vi "DPointGrayG3.vi"() -> ()   [LabVIEW 2011]
uses:
  <vilib>/vision/Image Controls.llb/IMAQ Image.ctl
  <vilib>/vision/driver/IMAQdx.llb/IMAQdx Camera Control Mode.ctl
  <vilib>/vision/driver/IMAQdx.llb/IMAQdx Attribute Type.ctl
  <vilib>/vision/driver/IMAQdx.llb/IMAQdx Buffer Number Mode.ctl
  <vilib>/vision/driver/IMAQdx.llb/IMAQdx Acquisition Mode.ctl
  <vilib>/vision/driver/NI_Vision_Acquisition_Software.lvlib
  National Instruments/LabVIEW 2011/resource/objmgr/imaqdx.rc
panel:
  out "String":string="cam0"
  out "binning":i32=1
  out "save all?":bool
  out "image":i32
  out "run":i32
  out "error":errorcluster
  # "Tested with GS3-U3-23S6\nIn M&A-Explorer:\nright click cam, Driver\nselect NI-IMAQdx ..USB3\nand test camera there\nexposure time is not correct\ndid not found the units 1µs?"
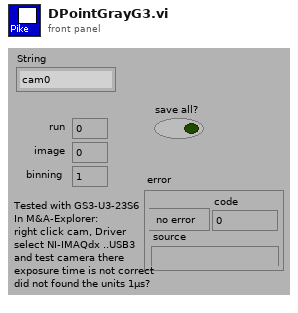
[diagram p1: front panel]
types:
  T1 = typedef "NI_Vision_Acquisition_Software.lvlib/IMAQdx Attribute Type.ctl" = enum32{"U32", "I64", "DBL", "String", "Enum", "Bool", "Command"}
  T2 = cluster{"Attribute Name":string, "Attribute Type":T1, "Value":string}[]
  T3 = cluster{"Attribute Type":T1, "Readable":bool, "Writable":bool, "Attribute Name":string, "Value":string}[]
  T4 = enum16{"None/#Datasets", "Clear", "TagValueOf#", "AddValues", "ReadValue", "ChangeValue", "Get all"}
  T5 = typedef "NI_Vision_Acquisition_Software.lvlib/IMAQdx Camera Control Mode.ctl" = enum32{"Controller", "Listener"}
  T6 = typedef "IMAQ Image.ctl" = refnum<image>
  T7 = cluster{"Type":u32, "Version":u32, "Flags":u32, "SerialNumberHigh":u32, "SerialNumberLow":u32, "BusType":u32, "InterfaceName":string, "VendorName":string, "ModelName":string, "CameraFileName":string, "CameraAttributeURL":string}[]
  T8 = typedef "IMAQdx.ctl" = refnum<k21>
  T9 = cluster{"Center":cluster{dbl, dbl}, "Rotate (rad)":dbl, "MirrorY":bool, "Scale":dbl}
  T10 = enum16{"status", "createIMAQ", "getIMAQ", "getNumber", "deleteIMAQ", "deleteAll", "MemoryUsage", "GetAccess", "DecreaseAccess", "ActualIndex", "ElementToNumber"}
  T11 = enum16{"status", "saveMeta", "getMeta", "deleteMeta", "deleteAll", "MemoryUsage"}
  T12 = typedef "NI_Vision_Acquisition_Software.lvlib/IMAQdx Buffer Number Mode.ctl" = enum32{"Next", "Last", "Buffer Number"}
  T13 = typedef "NI_Vision_Acquisition_Software.lvlib/IMAQdx Acquisition Mode.ctl" = enum32{"One Shot", "Continuous"}
  T14 = enum16{"status", "createIMAQ", "getIMAQ", "getNumber", "deleteIMAQ", "deleteAll", "MemoryUsage", "GetAccess", "DecreaseAccess", "ActualIndex"}
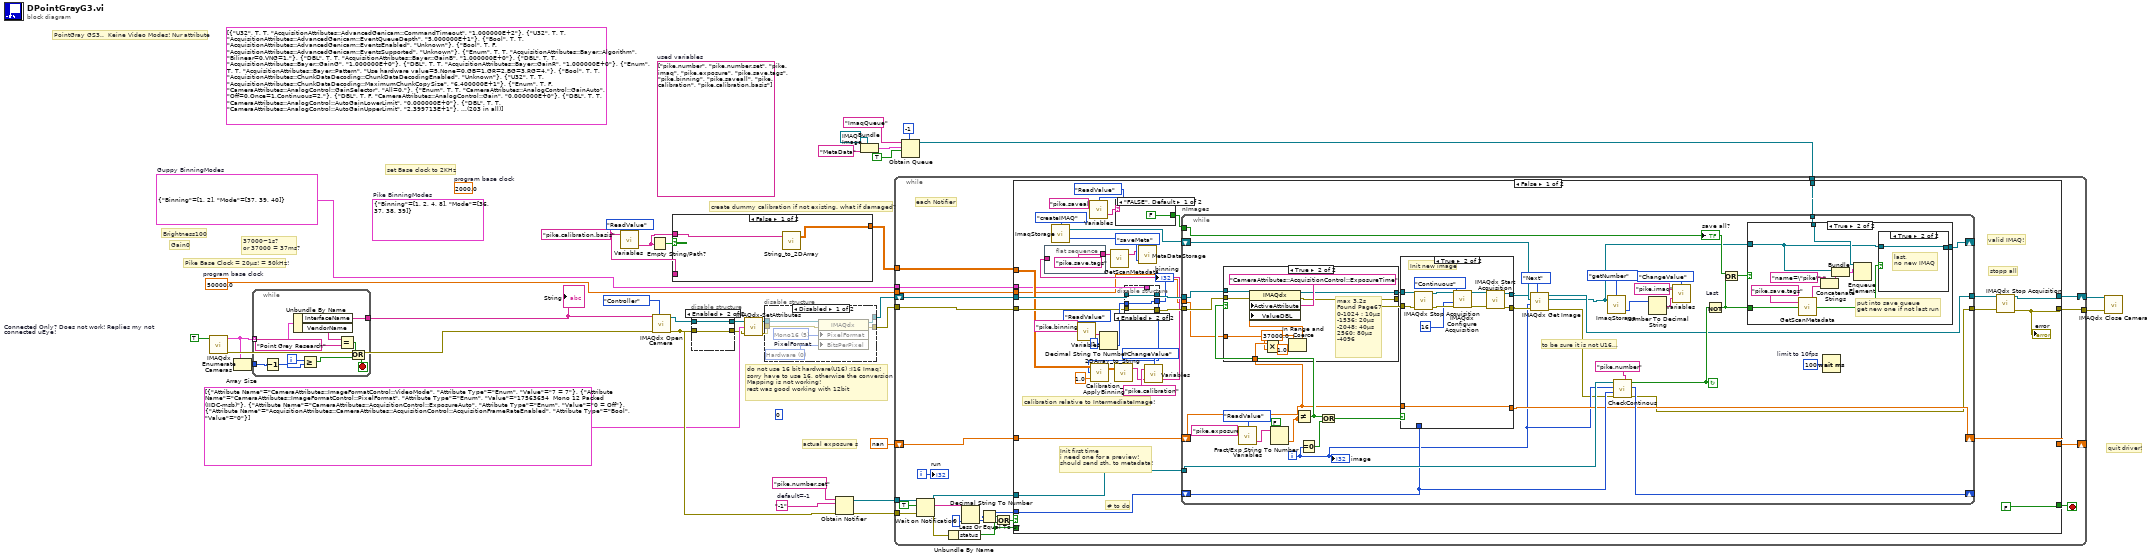
[diagram p0: block diagram]
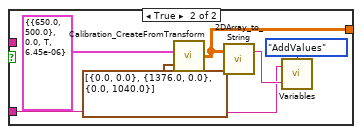
[diagram p3: hidden frame]
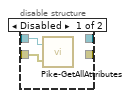
[diagram p4: hidden frame]
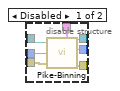
[diagram p5: hidden frame]
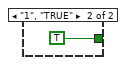
[diagram p6: hidden frame]
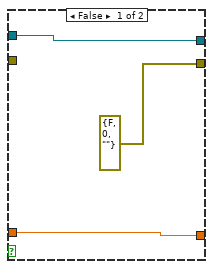
[diagram p8: hidden frame]
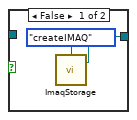
[diagram p10: hidden frame]
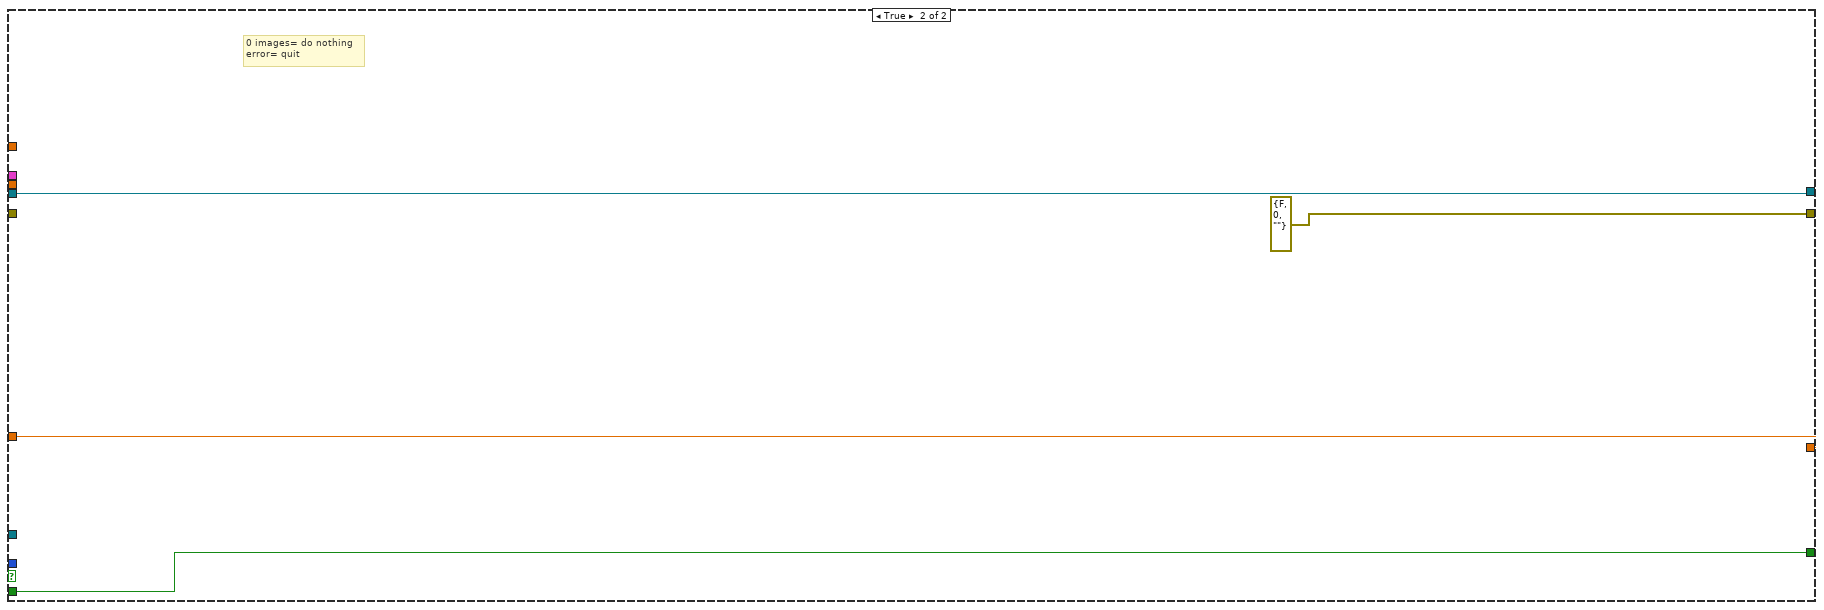
[diagram p11: hidden frame]
diagram:
  (unwired) u32 0 ("PixelFormat")
  (unwired) T3 [{"Attribute Type"=enum."U32", "Readable"=TRUE, "Writable"=TRUE, "Attribute Name"="AcquisitionAttributes::AdvancedGenicam::CommandTimeout", "Value"="1.000000E+2"}, {"Attribute Type"=enum."U32", "Readable"=TRUE, "Writable"=TRUE, "Attribute Name"="AcquisitionAttributes::AdvancedGenicam::EventQueueDepth", "Value"="5.000000E+1"}, {"Attribute Type"=enum."Bool", "Readable"=TRUE, "Writable"=TRUE, "Attribute Name"="AcquisitionAttributes::AdvancedGenicam::EventsEnabled", "Value"="Unknown"}, {"Attribute Type"=enum."Bool", "Readable"=TRUE, "Writable"=FALSE, "Attribute Name"="AcquisitionAttributes::AdvancedGenicam::EventsSupported", "Value"="Unknown"}, {"Attribute Type"=enum."Enum", "Readable"=TRUE, "Writable"=TRUE, "Attribute Name"="AcquisitionAttributes::Bayer::Algorithm", "Value"="Bilinear=0,VNG=1,"}, {"Attribute Type"=enum."DBL", "Readable"=TRUE, "Writable"=TRUE, "Attribute Name"="AcquisitionAttributes::Bayer::GainB", "Value"="1.000000E+0"}, {"Attribute Type"=enum."DBL", "Readable"=TRUE, "Writable"=TRUE, "Attribute Name"="AcquisitionAttributes::Bayer::GainG", "Value"="1.000000E+0"}, {"Attribute Type"=enum."DBL", "Readable"=TRUE, "Writable"=TRUE, "Attribute Name"="AcquisitionAttributes::Bayer::GainR", "Value"="1.000000E+0"}, {"Attribute Type"=enum."Enum", "Readable"=TRUE, "Writable"=TRUE, "Attribute Name"="AcquisitionAttributes::Bayer::Pattern", "Value"="Use hardware value=5,None=0,GB=1,GR=2,BG=3,RG=4,"}, {"Attribute Type"=enum."Bool", "Readable"=TRUE, "Writable"=TRUE, "Attribute Name"="AcquisitionAttributes::ChunkDataDecoding::ChunkDataDecodingEnabled", "Value"="Unknown"}, {"Attribute Type"=enum."U32", "Readable"=TRUE, "Writable"=TRUE, "Attribute Name"="AcquisitionAttributes::ChunkDataDecoding::MaximumChunkCopySize", "Value"="6.400000E+1"}, {"Attribute Type"=enum."Enum", "Readable"=TRUE, "Writable"=FALSE, "Attribute Name"="CameraAttributes::AnalogControl::GainSelector", "Value"="All=0,"}, {"Attribute Type"=enum."Enum", "Readable"=TRUE, "Writable"=TRUE, "Attribute Name"="CameraAttributes::AnalogControl::GainAuto", "Value"="Off=0,Once=1,Continuous=2,"}, {"Attribute Type"=enum."DBL", "Readable"=TRUE, "Writable"=FALSE, "Attribute Name"="CameraAttributes::AnalogControl::Gain", "Value"="0.000000E+0"}, {"Attribute Type"=enum."DBL", "Readable"=TRUE, "Writable"=TRUE, "Attribute Name"="CameraAttributes::AnalogControl::AutoGainLowerLimit", "Value"="0.000000E+0"}, {"Attribute Type"=enum."DBL", "Readable"=TRUE, "Writable"=TRUE, "Attribute Name"="CameraAttributes::AnalogControl::AutoGainUpperLimit", "Value"="2.399713E+1"}, {"Attribute Type"=enum."DBL", "Readable"=TRUE, "Writable"=TRUE, "Attribute Name"="CameraAttributes::AnalogControl::BlackLevel", "Value"="2.709961E+0"}, {"Attribute Type"=enum."Bool", "Readable"=TRUE, "Writable"=TRUE, "Attribute Name"="CameraAttributes::AnalogControl::BlackLevelEnabled", "Value"="Unknown"}, {"Attribute Type"=enum."DBL", "Readable"=TRUE, "Writable"=TRUE, "Attribute Name"="CameraAttributes::AnalogControl::Gamma", "Value"="1.250000E+0"}, {"Attribute Type"=enum."Bool", "Readable"=TRUE, "Writable"=TRUE, "Attribute Name"="CameraAttributes::AnalogControl::GammaEnabled", "Value"="Unknown"}, {"Attribute Type"=enum."I64", "Readable"=TRUE, "Writable"=FALSE, "Attribute Name"="CameraAttributes::AnalogControl::Sharpness", "Value"="1.534000E+3"}, {"Attribute Type"=enum."Bool", "Readable"=TRUE, "Writable"=TRUE, "Attribute Name"="CameraAttributes::AnalogControl::SharpnessEnabled", "Value"="Unknown"}, {"Attribute Type"=enum."Enum", "Readable"=TRUE, "Writable"=TRUE, "Attribute Name"="CameraAttributes::AnalogControl::SharpnessAuto", "Value"="Off=0,Continuous=2,"}, {"Attribute Type"=enum."Bool", "Readable"=FALSE, "Writable"=FALSE, "Attribute Name"="CameraAttributes::AnalogControl::HueEnabled", "Value"="Unknown"}, {"Attribute Type"=enum."Bool", "Readable"=FALSE, "Writable"=FALSE, "Attribute Name"="CameraAttributes::AnalogControl::SaturationEnabled", "Value"="Unknown"}, {"Attribute Type"=enum."String", "Readable"=TRUE, "Writable"=FALSE, "Attribute Name"="CameraAttributes::DeviceControl::DeviceVendorName", "Value"="Point Grey Research"}, {"Attribute Type"=enum."String", "Readable"=TRUE, "Writable"=FALSE, "Attribute Name"="CameraAttributes::DeviceControl::DeviceModelName", "Value"="Grasshopper3 GS3-U3-23S6M"}, {"Attribute Type"=enum."String", "Readable"=TRUE, "Writable"=FALSE, "Attribute Name"="CameraAttributes::DeviceControl::DeviceVersion", "Value"="FW:v2.7.3.00 FPGA:v2.02"}, {"Attribute Type"=enum."String", "Readable"=TRUE, "Writable"=FALSE, "Attribute Name"="CameraAttributes::DeviceControl::DeviceSerialNumber", "Value"="14120127"}, {"Attribute Type"=enum."String", "Readable"=TRUE, "Writable"=TRUE, "Attribute Name"="CameraAttributes::DeviceControl::DeviceUserID", "Value"=""}, {"Attribute Type"=enum."I64", "Readable"=TRUE, "Writable"=FALSE, "Attribute Name"="CameraAttributes::DeviceControl::DeviceGenCpVersionMajor", "Value"="1.000000E+0"}, {"Attribute Type"=enum."I64", "Readable"=TRUE, "Writable"=FALSE, "Attribute Name"="CameraAttributes::DeviceControl::DeviceGenCPVersionMinor", "Value"="0.000000E+0"}, {"Attribute Type"=enum."String", "Readable"=TRUE, "Writable"=FALSE, "Attribute Name"="CameraAttributes::DeviceControl::DeviceFamilyName", "Value"="GEN2-USB"}, {"Attribute Type"=enum."Bool", "Readable"=TRUE, "Writable"=FALSE, "Attribute Name"="CameraAttributes::DeviceControl::U3VDeviceCapability::UserNameAvailable", "Value"="Unknown"}, {"Attribute Type"=enum."Bool", "Readable"=TRUE, "Writable"=FALSE, "Attribute Name"="CameraAttributes::DeviceControl::U3VDeviceCapability::AccessPrivilegeAvailable", "Value"="Unknown"}, {"Attribute Type"=enum."Bool", "Readable"=TRUE, "Writable"=FALSE, "Attribute Name"="CameraAttributes::DeviceControl::U3VDeviceCapability::MessageChannelSupported", "Value"="Unknown"}, {"Attribute Type"=enum."Bool", "Readable"=TRUE, "Writable"=FALSE, "Attribute Name"="CameraAttributes::DeviceControl::U3VDeviceCapability::TimestampSupported", "Value"="Unknown"}, {"Attribute Type"=enum."I64", "Readable"=TRUE, "Writable"=FALSE, "Attribute Name"="CameraAttributes::DeviceControl::U3VDeviceCapability::StringEncoding", "Value"="0.000000E+0"}, {"Attribute Type"=enum."Bool", "Readable"=TRUE, "Writable"=FALSE, "Attribute Name"="CameraAttributes::DeviceControl::U3VDeviceCapability::FamilyRegisterAvailable", "Value"="Unknown"}, {"Attribute Type"=enum."Bool", "Readable"=TRUE, "Writable"=FALSE, "Attribute Name"="CameraAttributes::DeviceControl::U3VDeviceCapability::SBRMSupported", "Value"="Unknown"}, {"Attribute Type"=enum."Bool", "Readable"=TRUE, "Writable"=FALSE, "Attribute Name"="CameraAttributes::DeviceControl::U3VDeviceCapability::EndianessRegistersSupported", "Value"="Unknown"}, {"Attribute Type"=enum."Bool", "Readable"=TRUE, "Writable"=FALSE, "Attribute Name"="CameraAttributes::DeviceControl::U3VDeviceCapability::WrittenLengthFieldSupported", "Value"="Unknown"}, {"Attribute Type"=enum."I64", "Readable"=TRUE, "Writable"=FALSE, "Attribute Name"="CameraAttributes::DeviceControl::Timestamp", "Value"="0.000000E+0"}, {"Attribute Type"=enum."Command", "Readable"=FALSE, "Writable"=TRUE, "Attribute Name"="CameraAttributes::DeviceControl::TimestampLatch", "Value"="Unknown"}, {"Attribute Type"=enum."I64", "Readable"=TRUE, "Writable"=FALSE, "Attribute Name"="CameraAttributes::DeviceControl::TimestampIncrement", "Value"="1.250000E+5"}, {"Attribute Type"=enum."String", "Readable"=TRUE, "Writable"=FALSE, "Attribute Name"="CameraAttributes::DeviceControl::pgrSensorDescription", "Value"="Sony IMX174 (1/1.2\" Mono CMOS)"}, {"Attribute Type"=enum."String", "Readable"=TRUE, "Writable"=FALSE, "Attribute Name"="CameraAttributes::DeviceControl::DeviceSVNVersion", "Value"="FW:0 FPGA:0"}, {"Attribute Type"=enum."String", "Readable"=TRUE, "Writable"=FALSE, "Attribute Name"="CameraAttributes::DeviceControl::DeviceFirmwareVersion", "Value"="2.7.3.00"}, {"Attribute Type"=enum."Enum", "Readable"=TRUE, "Writable"=FALSE, "Attribute Name"="CameraAttributes::DeviceControl::DeviceScanType", "Value"="Areascan=0,"}, {"Attribute Type"=enum."DBL", "Readable"=TRUE, "Writable"=FALSE, "Attribute Name"="CameraAttributes::DeviceControl::DeviceTemperature", "Value"="4.785000E+1"}, {"Attribute Type"=enum."I64", "Readable"=TRUE, "Writable"=FALSE, "Attribute Name"="CameraAttributes::DeviceControl::pgrDeviceUptime", "Value"="9.150000E+2"}, {"Attribute Type"=enum."Enum", "Readable"=TRUE, "Writable"=TRUE, "Attribute Name"="CameraAttributes::DeviceControl::AutoFunctionAOIsControl", "Value"="Off=0,On=1,"}, {"Attribute Type"=enum."I64", "Readable"=FALSE, "Writable"=FALSE, "Attribute Name"="CameraAttributes::DeviceControl::AutoFunctionAOIWidth", "Value"="0.000000E+0"}, {"Attribute Type"=enum."I64", "Readable"=FALSE, "Writable"=FALSE, "Attribute Name"="CameraAttributes::DeviceControl::AutoFunctionAOIHeight", "Value"="0.000000E+0"}, {"Attribute Type"=enum."I64", "Readable"=FALSE, "Writable"=FALSE, "Attribute Name"="CameraAttributes::DeviceControl::AutoFunctionAOIOffsetX", "Value"="0.000000E+0"}, {"Attribute Type"=enum."I64", "Readable"=FALSE, "Writable"=FALSE, "Attribute Name"="CameraAttributes::DeviceControl::AutoFunctionAOIOffsetY", "Value"="0.000000E+0"}, {"Attribute Type"=enum."Enum", "Readable"=TRUE, "Writable"=TRUE, "Attribute Name"="CameraAttributes::DeviceControl::pgrDevicePowerSupplySelector", "Value"="External=0,LinkPower=1,5.0 Volts=2,Sensor Power=6,"}, {"Attribute Type"=enum."Enum", "Readable"=TRUE, "Writable"=FALSE, "Attribute Name"="CameraAttributes::DeviceControl::pgrPowerSourcePresent", "Value"="False=0,True=1,"}, {"Attribute Type"=enum."Enum", "Readable"=FALSE, "Writable"=FALSE, "Attribute Name"="CameraAttributes::DeviceControl::pgrPowerSupplyEnable", "Value"="False=0,True=1,"}, {"Attribute Type"=enum."DBL", "Readable"=TRUE, "Writable"=FALSE, "Attribute Name"="CameraAttributes::DeviceControl::pgrPowerSupplyVoltage", "Value"="0.000000E+0"}, {"Attribute Type"=enum."DBL", "Readable"=TRUE, "Writable"=FALSE, "Attribute Name"="CameraAttributes::DeviceControl::pgrPowerSupplyCurrent", "Value"="6.889992E-1"}, {"Attribute Type"=enum."I64", "Readable"=TRUE, "Writable"=FALSE, "Attribute Name"="CameraAttributes::DeviceControl::DeviceMaxThroughput", "Value"="3.041280E+8"}, {"Attribute Type"=enum."I64", "Readable"=TRUE, "Writable"=TRUE, "Attribute Name"="CameraAttributes::DeviceControl::DeviceLinkThroughputLimit", "Value"="3.041280E+8"}, {"Attribute Type"=enum."Enum", "Readable"=TRUE, "Writable"=TRUE, "Attribute Name"="CameraAttributes::AcquisitionControl::TriggerSelector", "Value"="Frame Start=0,Exposure Active=1,"}, {"Attribute Type"=enum."Enum", "Readable"=TRUE, "Writable"=TRUE, "Attribute Name"="CameraAttributes::AcquisitionControl::TriggerMode", "Value"="Off=0,On=1,"}, {"Attribute Type"=enum."Command", "Readable"=FALSE, "Writable"=FALSE, "Attribute Name"="CameraAttributes::AcquisitionControl::TriggerSoftware", "Value"="Unknown"}, {"Attribute Type"=enum."Enum", "Readable"=TRUE, "Writable"=TRUE, "Attribute Name"="CameraAttributes::AcquisitionControl::TriggerSource", "Value"="Software=7,Line 0=0,Line 2=2,Line 3=3,"}, {"Attribute Type"=enum."Enum", "Readable"=TRUE, "Writable"=TRUE, "Attribute Name"="CameraAttributes::AcquisitionControl::TriggerActivation", "Value"="Rising Edge=1,Falling Edge=0,"}, {"Attribute Type"=enum."DBL", "Readable"=TRUE, "Writable"=TRUE, "Attribute Name"="CameraAttributes::AcquisitionControl::TriggerDelay", "Value"="0.000000E+0"}, {"Attribute Type"=enum."Bool", "Readable"=TRUE, "Writable"=TRUE, "Attribute Name"="CameraAttributes::AcquisitionControl::TriggerDelayEnabled", "Value"="Unknown"}, {"Attribute Type"=enum."Enum", "Readable"=TRUE, "Writable"=TRUE, "Attribute Name"="CameraAttributes::AcquisitionControl::ExposureMode", "Value"="Timed=0,Trigger Width=1,"}, {"Attribute Type"=enum."Enum", "Readable"=TRUE, "Writable"=TRUE, "Attribute Name"="CameraAttributes::AcquisitionControl::ExposureAuto", "Value"="Off=0,Once=1,Continuous=2,"}, {"Attribute Type"=enum."DBL", "Readable"=TRUE, "Writable"=FALSE, "Attribute Name"="CameraAttributes::AcquisitionControl::ExposureTime", "Value"="2.435267E+3"}, {"Attribute Type"=enum."DBL", "Readable"=TRUE, "Writable"=TRUE, "Attribute Name"="CameraAttributes::AcquisitionControl::AutoExposureTimeLowerLimit", "Value"="9.119511E+0"}, {"Attribute Type"=enum."DBL", "Readable"=TRUE, "Writable"=TRUE, "Attribute Name"="CameraAttributes::AcquisitionControl::AutoExposureTimeUpperLimit", "Value"="1.152647E+4"}, {"Attribute Type"=enum."Enum", "Readable"=TRUE, "Writable"=TRUE, "Attribute Name"="CameraAttributes::AcquisitionControl::pgrExposureCompensationAuto", "Value"="Off=0,Once=1,Continuous=2,"}, {"Attribute Type"=enum."DBL", "Readable"=TRUE, "Writable"=FALSE, "Attribute Name"="CameraAttributes::AcquisitionControl::pgrExposureCompensation", "Value"="6.629639E-1"}, {"Attribute Type"=enum."DBL", "Readable"=TRUE, "Writable"=TRUE, "Attribute Name"="CameraAttributes::AcquisitionControl::pgrAutoExposureCompensationLowerLimit", "Value"="4.150391E-1"}, {"Attribute Type"=enum."DBL", "Readable"=TRUE, "Writable"=TRUE, "Attribute Name"="CameraAttributes::AcquisitionControl::pgrAutoExposureCompensationUpperLimit", "Value"="2.000000E+0"}, {"Attribute Type"=enum."Enum", "Readable"=TRUE, "Writable"=TRUE, "Attribute Name"="CameraAttributes::AcquisitionControl::AcquisitionMode", "Value"="Continuous=0,SingleFrame=1,MultiFrame=2,"}, {"Attribute Type"=enum."Enum", "Readable"=TRUE, "Writable"=TRUE, "Attribute Name"="CameraAttributes::AcquisitionControl::AcquisitionFrameRateAuto", "Value"="Off=0,Continuous=2,"}, {"Attribute Type"=enum."Bool", "Readable"=TRUE, "Writable"=TRUE, "Attribute Name"="CameraAttributes::AcquisitionControl::AcquisitionFrameRateEnabled", "Value"="Unknown"}, {"Attribute Type"=enum."DBL", "Readable"=TRUE, "Writable"=FALSE, "Attribute Name"="CameraAttributes::AcquisitionControl::AcquisitionFrameRate", "Value"="8.600000E+1"}, {"Attribute Type"=enum."I64", "Readable"=FALSE, "Writable"=FALSE, "Attribute Name"="CameraAttributes::AcquisitionControl::AcquisitionFrameCount", "Value"="0.000000E+0"}, {"Attribute Type"=enum."Enum", "Readable"=TRUE, "Writable"=TRUE, "Attribute Name"="CameraAttributes::ImageFormatControl::PixelFormat", "Value"="Mono 8=17301505,Mono 12 Packed (IIDC-msb)=17563654,Mono 12 Packed=17563719,Mono 16=17825799,"}, {"Attribute Type"=enum."Bool", "Readable"=TRUE, "Writable"=TRUE, "Attribute Name"="CameraAttributes::ImageFormatControl::OnBoardColorProcessEnabled", "Value"="Unknown"}, {"Attribute Type"=enum."I64", "Readable"=TRUE, "Writable"=TRUE, "Attribute Name"="CameraAttributes::ImageFormatControl::Width", "Value"="1.920000E+3"}, {"Attribute Type"=enum."I64", "Readable"=TRUE, "Writable"=TRUE, "Attribute Name"="CameraAttributes::ImageFormatControl::Height", "Value"="1.200000E+3"}, {"Attribute Type"=enum."I64", "Readable"=TRUE, "Writable"=TRUE, "Attribute Name"="CameraAttributes::ImageFormatControl::OffsetX", "Value"="0.000000E+0"}, {"Attribute Type"=enum."I64", "Readable"=TRUE, "Writable"=TRUE, "Attribute Name"="CameraAttributes::ImageFormatControl::OffsetY", "Value"="0.000000E+0"}, {"Attribute Type"=enum."I64", "Readable"=TRUE, "Writable"=FALSE, "Attribute Name"="CameraAttributes::ImageFormatControl::SensorWidth", "Value"="1.920000E+3"}, {"Attribute Type"=enum."I64", "Readable"=TRUE, "Writable"=FALSE, "Attribute Name"="CameraAttributes::ImageFormatControl::SensorHeight", "Value"="1.200000E+3"}, {"Attribute Type"=enum."I64", "Readable"=TRUE, "Writable"=FALSE, "Attribute Name"="CameraAttributes::ImageFormatControl::WidthMax", "Value"="1.920000E+3"}, {"Attribute Type"=enum."I64", "Readable"=TRUE, "Writable"=FALSE, "Attribute Name"="CameraAttributes::ImageFormatControl::HeightMax", "Value"="1.200000E+3"}, {"Attribute Type"=enum."Enum", "Readable"=TRUE, "Writable"=TRUE, "Attribute Name"="CameraAttributes::ImageFormatControl::VideoMode", "Value"="0=0,1=1,7=7,"}, {"Attribute Type"=enum."I64", "Readable"=TRUE, "Writable"=FALSE, "Attribute Name"="CameraAttributes::ImageFormatControl::BinningHorizontal", "Value"="1.000000E+0"}, {"Attribute Type"=enum."I64", "Readable"=TRUE, "Writable"=TRUE, "Attribute Name"="CameraAttributes::ImageFormatControl::BinningVertical", "Value"="1.000000E+0"}, {"Attribute Type"=enum."Bool", "Readable"=TRUE, "Writable"=TRUE, "Attribute Name"="CameraAttributes::ImageFormatControl::ReverseX", "Value"="Unknown"}, {"Attribute Type"=enum."Enum", "Readable"=TRUE, "Writable"=FALSE, "Attribute Name"="CameraAttributes::ImageFormatControl::PixelSize", "Value"="8 Bits/Pixel=8,10 Bits/Pixel=10,12 Bits/Pixel=12,16 Bits/Pixel=16,24 Bits/Pixel=24,32 Bits/Pixel=32,"}, {"Attribute Type"=enum."Enum", "Readable"=TRUE, "Writable"=FALSE, "Attribute Name"="CameraAttributes::ImageFormatControl::PixelColorFilter", "Value"="BayerRG=0,BayerGB=1,BayerGR=2,BayerBG=3,None=255,"}, {"Attribute Type"=enum."I64", "Readable"=TRUE, "Writable"=FALSE, "Attribute Name"="CameraAttributes::ImageFormatControl::PixelDynamicRangeMin", "Value"="0.000000E+0"}, {"Attribute Type"=enum."I64", "Readable"=TRUE, "Writable"=FALSE, "Attribute Name"="CameraAttributes::ImageFormatControl::PixelDynamicRangeMax", "Value"="0.000000E+0"}, {"Attribute Type"=enum."Enum", "Readable"=TRUE, "Writable"=TRUE, "Attribute Name"="CameraAttributes::ImageFormatControl::TestPattern", "Value"="Off=0,Test Image 1=1,Test Image 2=2,"}, {"Attribute Type"=enum."Enum", "Readable"=TRUE, "Writable"=FALSE, "Attribute Name"="CameraAttributes::ImageFormatControl::PixelDefectControl::pgrDefectPixelCorrectionType", "Value"="FPGA Correction=0,Sensor Correction=1,"}, {"Attribute Type"=enum."Bool", "Readable"=TRUE, "Writable"=TRUE, "Attribute Name"="CameraAttributes::ImageFormatControl::PixelDefectControl::pgrDefectPixelCorrectionEnable", "Value"="Unknown"}, {"Attribute Type"=enum."Enum", "Readable"=TRUE, "Writable"=TRUE, "Attribute Name"="CameraAttributes::ImageFormatControl::PixelDefectControl::pgrDefectPixelCorrectionTestMode", "Value"="Off=0,On=1,"}, {"Attribute Type"=enum."I64", "Readable"=TRUE, "Writable"=TRUE, "Attribute Name"="CameraAttributes::ImageFormatControl::PixelDefectControl::pgrCurrentCorrectedPixelCount", "Value"="6.000000E+0"}, {"Attribute Type"=enum."I64", "Readable"=TRUE, "Writable"=TRUE, "Attribute Name"="CameraAttributes::ImageFormatControl::PixelDefectControl::pgrCurrentCorrectedPixelIndex", "Value"="0.000000E+0"}, {"Attribute Type"=enum."I64", "Readable"=TRUE, "Writable"=TRUE, "Attribute Name"="CameraAttributes::ImageFormatControl::PixelDefectControl::pgrCurrentCorrectedPixelOffsetX", "Value"="1.151000E+3"}, {"Attribute Type"=enum."I64", "Readable"=TRUE, "Writable"=TRUE, "Attribute Name"="CameraAttributes::ImageFormatControl::PixelDefectControl::pgrCurrentCorrectedPixelOffsetY", "Value"="5.900000E+1"}, {"Attribute Type"=enum."Command", "Readable"=FALSE, "Writable"=TRUE, "Attribute Name"="CameraAttributes::ImageFormatControl::PixelDefectControl::pgrCurrentCorrectedPixelSave", "Value"="Unknown"}, {"Attribute Type"=enum."I64", "Readable"=TRUE, "Writable"=FALSE, "Attribute Name"="CameraAttributes::UserSetControl::UserSetCurrent", "Value"="0.000000E+0"}, {"Attribute Type"=enum."Enum", "Readable"=TRUE, "Writable"=TRUE, "Attribute Name"="CameraAttributes::UserSetControl::UserSetSelector", "Value"="Default=0,User Set 1=1,User Set 2=2,"}, {"Attribute Type"=enum."Command", "Readable"=FALSE, "Writable"=TRUE, "Attribute Name"="CameraAttributes::UserSetControl::UserSetLoad", "Value"="Unknown"}, {"Attribute Type"=enum."Command", "Readable"=FALSE, "Writable"=TRUE, "Attribute Name"="CameraAttributes::UserSetControl::UserSetSave", "Value"="Unknown"}, {"Attribute Type"=enum."Enum", "Readable"=TRUE, "Writable"=TRUE, "Attribute Name"="CameraAttributes::UserSetControl::UserSetDefault", "Value"="Default=0,User Set 1=1,User Set 2=2,"}, {"Attribute Type"=enum."I64", "Readable"=TRUE, "Writable"=FALSE, "Attribute Name"="CameraAttributes::DataFlashControl::DataFlashPageSize", "Value"="2.560000E+2"}, {"Attribute Type"=enum."I64", "Readable"=TRUE, "Writable"=FALSE, "Attribute Name"="CameraAttributes::DataFlashControl::DataFlashPageCount", "Value"="8.192000E+3"}, {"Attribute Type"=enum."I64", "Readable"=TRUE, "Writable"=TRUE, "Attribute Name"="CameraAttributes::DataFlashControl::ActivePageNumber", "Value"="0.000000E+0"}, {"Attribute Type"=enum."I64", "Readable"=TRUE, "Writable"=TRUE, "Attribute Name"="CameraAttributes::DataFlashControl::ActivePageOffset", "Value"="0.000000E+0"}, {"Attribute Type"=enum."I64", "Readable"=TRUE, "Writable"=TRUE, "Attribute Name"="CameraAttributes::DataFlashControl::ActivePageValue", "Value"="1.129859E+9"}, {"Attribute Type"=enum."Command", "Readable"=FALSE, "Writable"=TRUE, "Attribute Name"="CameraAttributes::DataFlashControl::ActivePageSave", "Value"="Unknown"}, {"Attribute Type"=enum."Enum", "Readable"=TRUE, "Writable"=TRUE, "Attribute Name"="CameraAttributes::DigitalIOControl::LineSelector", "Value"="Line 0=0,Line 1=1,Line 2=2,Line 3=3,"}, {"Attribute Type"=enum."Enum", "Readable"=TRUE, "Writable"=TRUE, "Attribute Name"="CameraAttributes::DigitalIOControl::LineMode", "Value"="Input=0,Trigger=2,"}, {"Attribute Type"=enum."Enum", "Readable"=FALSE, "Writable"=FALSE, "Attribute Name"="CameraAttributes::DigitalIOControl::LineSource", "Value"="ExposureActive=0,ExternalTriggerActive=1,"}, {"Attribute Type"=enum."Bool", "Readable"=FALSE, "Writable"=FALSE, "Attribute Name"="CameraAttributes::DigitalIOControl::LineInverter", "Value"="Unknown"}, {"Attribute Type"=enum."Bool", "Readable"=FALSE, "Writable"=FALSE, "Attribute Name"="CameraAttributes::DigitalIOControl::StrobeEnabled", "Value"="Unknown"}, {"Attribute Type"=enum."DBL", "Readable"=FALSE, "Writable"=FALSE, "Attribute Name"="CameraAttributes::DigitalIOControl::StrobeDelay", "Value"="0.000000E+0"}, {"Attribute Type"=enum."DBL", "Readable"=FALSE, "Writable"=FALSE, "Attribute Name"="CameraAttributes::DigitalIOControl::StrobeDuration", "Value"="0.000000E+0"}, {"Attribute Type"=enum."Bool", "Readable"=FALSE, "Writable"=FALSE, "Attribute Name"="CameraAttributes::DigitalIOControl::UserOutputValue", "Value"="Unknown"}, {"Attribute Type"=enum."I64", "Readable"=TRUE, "Writable"=TRUE, "Attribute Name"="CameraAttributes::DigitalIOControl::LineDebouncerTimeRaw", "Value"="0.000000E+0"}, {"Attribute Type"=enum."Bool", "Readable"=TRUE, "Writable"=FALSE, "Attribute Name"="CameraAttributes::DigitalIOControl::LineStatus", "Value"="Unknown"}, {"Attribute Type"=enum."I64", "Readable"=TRUE, "Writable"=FALSE, "Attribute Name"="CameraAttributes::DigitalIOControl::LineStatusAll", "Value"="1.400000E+1"}, {"Attribute Type"=enum."I64", "Readable"=TRUE, "Writable"=TRUE, "Attribute Name"="CameraAttributes::TransportLayerControl::U3VMessageChannelID", "Value"="0.000000E+0"}, {"Attribute Type"=enum."I64", "Readable"=TRUE, "Writable"=FALSE, "Attribute Name"="CameraAttributes::TransportLayerControl::U3VVersionMajor", "Value"="1.000000E+0"}, {"Attribute Type"=enum."I64", "Readable"=TRUE, "Writable"=FALSE, "Attribute Name"="CameraAttributes::TransportLayerControl::U3VVersionMinor", "Value"="0.000000E+0"}, {"Attribute Type"=enum."I64", "Readable"=TRUE, "Writable"=FALSE, "Attribute Name"="CameraAttributes::TransportLayerControl::U3VCPCapability", "Value"="0.000000E+0"}, {"Attribute Type"=enum."Bool", "Readable"=TRUE, "Writable"=FALSE, "Attribute Name"="CameraAttributes::TransportLayerControl::U3VCPSIRMAvailable", "Value"="Unknown"}, {"Attribute Type"=enum."Bool", "Readable"=TRUE, "Writable"=FALSE, "Attribute Name"="CameraAttributes::TransportLayerControl::U3VCPEIRMAvailable", "Value"="Unknown"}, {"Attribute Type"=enum."Bool", "Readable"=TRUE, "Writable"=FALSE, "Attribute Name"="CameraAttributes::TransportLayerControl::U3VCPIIDC2Available", "Value"="Unknown"}, {"Attribute Type"=enum."I64", "Readable"=TRUE, "Writable"=FALSE, "Attribute Name"="CameraAttributes::TransportLayerControl::U3VMaxCommandTransferLength", "Value"="1.024000E+3"}, {"Attribute Type"=enum."I64", "Readable"=TRUE, "Writable"=FALSE, "Attribute Name"="CameraAttributes::TransportLayerControl::U3VMaxAcknowledgeTransferLength", "Value"="1.024000E+3"}, {"Attribute Type"=enum."I64", "Readable"=TRUE, "Writable"=FALSE, "Attribute Name"="CameraAttributes::TransportLayerControl::U3VNumberOfStreamChannels", "Value"="1.000000E+0"}, {"Attribute Type"=enum."Enum", "Readable"=TRUE, "Writable"=FALSE, "Attribute Name"="CameraAttributes::TransportLayerControl::U3VCurrentSpeed", "Value"="Low Speed=0,Full Speed=1,High Speed=2,Super Speed=3,"}, {"Attribute Type"=enum."I64", "Readable"=TRUE, "Writable"=FALSE, "Attribute Name"="CameraAttributes::TransportLayerControl::PayloadSize", "Value"="3.456000E+6"}, {"Attribute Type"=enum."I64", "Readable"=TRUE, "Writable"=FALSE, "Attribute Name"="CameraAttributes::TransportLayerControl::TransmitFailureCount", "Value"="0.000000E+0"}, {"Attribute Type"=enum."Command", "Readable"=FALSE, "Writable"=TRUE, "Attribute Name"="CameraAttributes::TransportLayerControl::TransmitFailureCountReset", "Value"="Unknown"}, {"Attribute Type"=enum."I64", "Readable"=TRUE, "Writable"=FALSE, "Attribute Name"="CameraAttributes::TransportLayerControl::USB3LinkRecoveryCount", "Value"="0.000000E+0"}, {"Attribute Type"=enum."Bool", "Readable"=TRUE, "Writable"=TRUE, "Attribute Name"="CameraAttributes::ChunkDataControl::ChunkModeActive", "Value"="Unknown"}, {"Attribute Type"=enum."Enum", "Readable"=TRUE, "Writable"=TRUE, "Attribute Name"="CameraAttributes::ChunkDataControl::ChunkSelector", "Value"="Image CRC=1,Frame Counter=2,Offset X=3,Offset Y=4,Width=5,Height=6,Exposure Time=7,Gain=8,Black Level=9,"}, {"Attribute Type"=enum."Bool", "Readable"=TRUE, "Writable"=TRUE, "Attribute Name"="CameraAttributes::ChunkDataControl::ChunkEnable", "Value"="Unknown"}, {"Attribute Type"=enum."I64", "Readable"=FALSE, "Writable"=FALSE, "Attribute Name"="CameraAttributes::ChunkData::ChunkCRC", "Value"="0.000000E+0"}, {"Attribute Type"=enum."I64", "Readable"=FALSE, "Writable"=FALSE, "Attribute Name"="CameraAttributes::ChunkData::ChunkFrameCounter", "Value"="0.000000E+0"}, {"Attribute Type"=enum."I64", "Readable"=FALSE, "Writable"=FALSE, "Attribute Name"="CameraAttributes::ChunkData::ChunkOffsetX", "Value"="0.000000E+0"}, {"Attribute Type"=enum."I64", "Readable"=FALSE, "Writable"=FALSE, "Attribute Name"="CameraAttributes::ChunkData::ChunkOffsetY", "Value"="0.000000E+0"}, {"Attribute Type"=enum."I64", "Readable"=FALSE, "Writable"=FALSE, "Attribute Name"="CameraAttributes::ChunkData::ChunkWidth", "Value"="0.000000E+0"}, {"Attribute Type"=enum."I64", "Readable"=FALSE, "Writable"=FALSE, "Attribute Name"="CameraAttributes::ChunkData::ChunkHeight", "Value"="0.000000E+0"}, {"Attribute Type"=enum."DBL", "Readable"=FALSE, "Writable"=FALSE, "Attribute Name"="CameraAttributes::ChunkData::ChunkExposureTime", "Value"="0.000000E+0"}, {"Attribute Type"=enum."DBL", "Readable"=FALSE, "Writable"=FALSE, "Attribute Name"="CameraAttributes::ChunkData::ChunkGain", "Value"="0.000000E+0"}, {"Attribute Type"=enum."DBL", "Readable"=FALSE, "Writable"=FALSE, "Attribute Name"="CameraAttributes::ChunkData::ChunkBlackLevel", "Value"="0.000000E+0"}, {"Attribute Type"=enum."Enum", "Readable"=TRUE, "Writable"=TRUE, "Attribute Name"="CameraAttributes::EventControl::EventSelector", "Value"="Acquisition Start=40000,Acquisition End=40001,Exposure Start=40002,Exposure End=40003,"}, {"Attribute Type"=enum."Enum", "Readable"=TRUE, "Writable"=TRUE, "Attribute Name"="CameraAttributes::EventControl::EventNotification", "Value"="On=1,Off=0,"}, {"Attribute Type"=enum."I64", "Readable"=FALSE, "Writable"=FALSE, "Attribute Name"="CameraAttributes::EventControl::EventAcquisitionStartData::EventAcquisitionStart", "Value"="0.000000E+0"}, {"Attribute Type"=enum."I64", "Readable"=FALSE, "Writable"=FALSE, "Attribute Name"="CameraAttributes::EventControl::EventAcquisitionStartData::EventAcquisitionStartTimestamp", "Value"="0.000000E+0"}, {"Attribute Type"=enum."I64", "Readable"=FALSE, "Writable"=FALSE, "Attribute Name"="CameraAttributes::EventControl::EventAcquisitionStartData::EventAcquisitionStartFrameID", "Value"="0.000000E+0"}, {"Attribute Type"=enum."I64", "Readable"=FALSE, "Writable"=FALSE, "Attribute Name"="CameraAttributes::EventControl::EventAcquisitionEndData::EventAcquisitionEnd", "Value"="0.000000E+0"}, {"Attribute Type"=enum."I64", "Readable"=FALSE, "Writable"=FALSE, "Attribute Name"="CameraAttributes::EventControl::EventAcquisitionEndData::EventAcquisitionEndTimestamp", "Value"="0.000000E+0"}, {"Attribute Type"=enum."I64", "Readable"=FALSE, "Writable"=FALSE, "Attribute Name"="CameraAttributes::EventControl::EventAcquisitionEndData::EventAcquisitionEndFrameID", "Value"="0.000000E+0"}, {"Attribute Type"=enum."I64", "Readable"=FALSE, "Writable"=FALSE, "Attribute Name"="CameraAttributes::EventControl::EventExposureStartData::EventExposureStart", "Value"="0.000000E+0"}, {"Attribute Type"=enum."I64", "Readable"=FALSE, "Writable"=FALSE, "Attribute Name"="CameraAttributes::EventControl::EventExposureStartData::EventExposureStartTimestamp", "Value"="0.000000E+0"}, {"Attribute Type"=enum."I64", "Readable"=FALSE, "Writable"=FALSE, "Attribute Name"="CameraAttributes::EventControl::EventExposureStartData::EventExposureStartFrameID", "Value"="0.000000E+0"}, {"Attribute Type"=enum."I64", "Readable"=FALSE, "Writable"=FALSE, "Attribute Name"="CameraAttributes::EventControl::EventExposureEndData::EventExposureEnd", "Value"="0.000000E+0"}, {"Attribute Type"=enum."I64", "Readable"=FALSE, "Writable"=FALSE, "Attribute Name"="CameraAttributes::EventControl::EventExposureEndData::EventExposureEndTimestamp", "Value"="0.000000E+0"}, {"Attribute Type"=enum."I64", "Readable"=FALSE, "Writable"=FALSE, "Attribute Name"="CameraAttributes::EventControl::EventExposureEndData::EventExposureEndFrameID", "Value"="0.000000E+0"}, {"Attribute Type"=enum."Command", "Readable"=FALSE, "Writable"=TRUE, "Attribute Name"="CameraAttributes::EventControl::TriggerEventTest", "Value"="Unknown"}, {"Attribute Type"=enum."I64", "Readable"=FALSE, "Writable"=FALSE, "Attribute Name"="CameraAttributes::EventControl::EventTestData::EventTest", "Value"="0.000000E+0"}, {"Attribute Type"=enum."I64", "Readable"=FALSE, "Writable"=FALSE, "Attribute Name"="CameraAttributes::EventControl::EventTestData::EventTestTimestamp", "Value"="0.000000E+0"}, {"Attribute Type"=enum."I64", "Readable"=FALSE, "Writable"=FALSE, "Attribute Name"="CameraAttributes::EventControl::EventTestData::EventTestFrameID", "Value"="0.000000E+0"}, {"Attribute Type"=enum."Enum", "Readable"=TRUE, "Writable"=TRUE, "Attribute Name"="AcquisitionAttributes::BitsPerPixel", "Value"="Use hardware value=0,10-bit=10,12-bit=12,14-bit=14,16-bit=16,"}, {"Attribute Type"=enum."Enum", "Readable"=TRUE, "Writable"=TRUE, "Attribute Name"="AcquisitionAttributes::ImageDecoderCopyMode", "Value"="Auto=0,Always=1,Never=2,"}, {"Attribute Type"=enum."Enum", "Readable"=TRUE, "Writable"=TRUE, "Attribute Name"="AcquisitionAttributes::IncompleteBufferMode", "Value"="Ignore=0,Fail=1,"}, {"Attribute Type"=enum."Enum", "Readable"=TRUE, "Writable"=TRUE, "Attribute Name"="AcquisitionAttributes::OutputImageType", "Value"="Auto=2147483647,Grayscale (U8)=0,Grayscale (I16)=1,Grayscale (U16)=7,RGB (U32)=4,RGB (U64)=6,"}, {"Attribute Type"=enum."Enum", "Readable"=TRUE, "Writable"=TRUE, "Attribute Name"="AcquisitionAttributes::OverwriteMode", "Value"="Get Oldest=0,Fail=2,Get Newest=3,"}, {"Attribute Type"=enum."Enum", "Readable"=TRUE, "Writable"=TRUE, "Attribute Name"="AcquisitionAttributes::ReceiveTimestampMode", "Value"="None=0,Tick Count=1,System Time=2,"}, {"Attribute Type"=enum."Bool", "Readable"=TRUE, "Writable"=TRUE, "Attribute Name"="AcquisitionAttributes::ShiftPixelBits", "Value"="Unknown"}, {"Attribute Type"=enum."Bool", "Readable"=TRUE, "Writable"=TRUE, "Attribute Name"="AcquisitionAttributes::SwapPixelBytes", "Value"="Unknown"}, {"Attribute Type"=enum."U32", "Readable"=TRUE, "Writable"=TRUE, "Attribute Name"="AcquisitionAttributes::Timeout", "Value"="5.000000E+3"}, {"Attribute Type"=enum."U32", "Readable"=TRUE, "Writable"=FALSE, "Attribute Name"="CameraInformation::BaseAddress", "Value"="0.000000E+0"}, {"Attribute Type"=enum."Enum", "Readable"=TRUE, "Writable"=FALSE, "Attribute Name"="CameraInformation::BusType", "Value"="FireWire=825440564,Ethernet=1768977972,Simulator=544434541,DirectShow=1685284983,IP=1230005101,SmartCamera2=1396924722,USB3 Vision=1431519795,UVC=1431716640,"}, {"Attribute Type"=enum."String", "Readable"=TRUE, "Writable"=FALSE, "Attribute Name"="CameraInformation::ModelName", "Value"="Grasshopper3 GS3-U3-23S6M"}, {"Attribute Type"=enum."String", "Readable"=TRUE, "Writable"=FALSE, "Attribute Name"="CameraInformation::PrimaryURLString", "Value"="Local:Point Grey Research_GEN2-USB_Grasshopper3 GS3-U3-23S6M_FW_v2.7.3.00 FPGA_v2.02_95785afa5ee09562316bc701b412815e5437e6de.zip;00000000fffd0040;0000000000006d52"}, {"Attribute Type"=enum."String", "Readable"=TRUE, "Writable"=FALSE, "Attribute Name"="CameraInformation::SecondaryURLString", "Value"=""}, {"Attribute Type"=enum."U32", "Readable"=TRUE, "Writable"=FALSE, "Attribute Name"="CameraInformation::SerialNumberHigh", "Value"="7.696000E+3"}, {"Attribute Type"=enum."U32", "Readable"=TRUE, "Writable"=FALSE, "Attribute Name"="CameraInformation::SerialNumberLow", "Value"="1.412013E+7"}, {"Attribute Type"=enum."Enum", "Readable"=TRUE, "Writable"=FALSE, "Attribute Name"="CameraInformation::USBConnectionSpeed", "Value"="Low-Speed (USB 2.0)=1,Full-Speed (USB 2.0)=2,Hi-Speed (USB 2.0)=4,SuperSpeed (USB 3.0)=8,"}, {"Attribute Type"=enum."String", "Readable"=TRUE, "Writable"=FALSE, "Attribute Name"="CameraInformation::VendorName", "Value"="Point Grey Research"}, {"Attribute Type"=enum."Bool", "Readable"=TRUE, "Writable"=FALSE, "Attribute Name"="StatusInformation::AcqInProgress", "Value"="Unknown"}, {"Attribute Type"=enum."I64", "Readable"=TRUE, "Writable"=FALSE, "Attribute Name"="StatusInformation::HandledEventCount", "Value"="0.000000E+0"}, {"Attribute Type"=enum."I64", "Readable"=TRUE, "Writable"=FALSE, "Attribute Name"="StatusInformation::IncompleteBufferCount", "Value"="0.000000E+0"}, {"Attribute Type"=enum."I64", "Readable"=TRUE, "Writable"=FALSE, "Attribute Name"="StatusInformation::LastBufferCount", "Value"="0.000000E+0"}, {"Attribute Type"=enum."U32", "Readable"=TRUE, "Writable"=FALSE, "Attribute Name"="StatusInformation::LastBufferNumber", "Value"="4.294967E+9"}, {"Attribute Type"=enum."I64", "Readable"=TRUE, "Writable"=FALSE, "Attribute Name"="StatusInformation::LostBufferCount", "Value"="0.000000E+0"}, {"Attribute Type"=enum."I64", "Readable"=TRUE, "Writable"=FALSE, "Attribute Name"="StatusInformation::LostEventCount", "Value"="0.000000E+0"}] ("Array")
  w6 = 50000.0  # program base clock
  (unwired) 2000.0  # program base clock
  w7 = cluster{"Binning":i32[], "Mode":u16[]} {"Binning"=[1, 2], "Mode"=[37, 39, 40]}  # Guppy BinningModes
  (unwired) cluster{"Binning":i32[], "Mode":u16[]} {"Binning"=[1, 2, 4, 8], "Mode"=[36, 37, 38, 39]}  # Pike BinningModes
  w13 = TRUE  # Connected Only? Does not work! Replies my not connected uEye!
  w15 = "pike.calibration.basis" ("Tag in")
  (unwired) string[] ["pike.number", "pike.number.set", "pike.imaq", "pike.exposure", "pike.save.tags", "pike.binning", "pike.saveall", "pike.calibration", "pike.calibration.basis"]  # used variables
  w28 = "-1"  # default=-1
  # "37000~1s?\nor 37000 = 37ms?"
  # "PointGray GS3..  Keine Video Modes! Nur attribute"
  # "Pike Base Clock = 20µs! = 50kHz!"
  # "set Base clock to 2KHz"
  # "Gain0"
  # "Brightness100"
  # "create dummy calibration if not existing. what if damaged?"
  # "do not use 16 bit hardware(U16) :I16 Imaq!\nsorry have to use 16, otherwise the conversion\nMapping is not working! \nrest was good working with 12bit"
  # "actual exposure s"
  # "quit driver!"
  n1 = call <vilib>:"IMAQdx Enumerate Cameras.vi"("Connected Only? (Yes)"=w13) -> ("error out"=w11:errorcluster, "Camera Information Array"=w10:T7)  [unwired: 1 in, 8 out]
  n2 = Array Size(array=w10) -> (size(s)=w9:i32)
  n3 = Decrement(x=w9) -> (x-1=w8:i32)
  n4 = while {
    tunnel: w10 -> [w45] mode=indexing
    tunnel: [w46] -> w12
    tunnel: w8 -> [w40]
    i -> [w41]
    stop <- w39 stop-if-true
    n5 = Unbundle By Name(w45) -> ("InterfaceName"=w46:string, "VendorName"=w44:string)
    n6 = Greater Or Equal?(x=w41, y=w40) -> (x >= y?=w38:bool)
    n7 = Equal?(x=w44, y="Point Grey Research") -> (x = y?=w42:bool)
    n8 = Or(x=w42, y=w38) -> (x .or. y?=w39:bool)
  }
  "String" <- w12
  n9 = call "Variables.vi"("Tag in"=w15, "Command"=T4."ReadValue") -> ("value out"=w14:string)  [unwired: 1 in, 2 out]
  n10 = Empty String/Path?(string/path=w14) -> (empty?=w17:bool)
  n11 = call <vilib>:"IMAQdx Open Camera.vi"("Camera Control Mode"=IMAQdx_Camera_Control_Mode."Controller", "error in"=w11, "Session In"=w12) -> ("error out"=w18:errorcluster, "Session Out"=w20:T8)  [unwired: 7 out]
  n12 = case shown="False" w17 {
    tunnel: w14 -> [w47 _]
    tunnel: [w48 w54] -> w16
    tunnel: w15 -> [_ w51]
    frame False {
      n13 = call "String_to_2DArray.vi"("String"=w47) -> ("Array"=w48:dbl[][])  [unwired: 3 in, 1 out]
    }
    frame True {
      n14 = call "Calibration_CreateFromTransform.vi"("sample points"=cluster{dbl, dbl}[] [{0.0, 0.0}, {1376.0, 0.0}, {0.0, 1040.0}], "Transform (Center first)"=T9 {"Center"={650.0, 500.0}, "Rotate (rad)"=0.0, "MirrorY"=TRUE, "Scale"=6.45e-06}) -> ("CalibrationCoordinates: x,x',y,y'..."=w54:dbl[][])
      n15 = call "2DArray_to_String.vi"("Array"=w54) -> ("String 1"=w52:string)  [unwired: 3 in, 1 out]
      n16 = call "Variables.vi"("value"=w52, "Tag in"=w51, "Command"=T4."AddValues") -> ()  [unwired: 3 out]
    }
  }
  n17 = disable-structure shown="Enabled" {
    disable-tunnel: w20 -> [w56 w58]
    disable-tunnel: w18 -> [w55 w57]
    disable-tunnel: [_ w58] -> w4
    disable-tunnel: [_ w57] -> w2
    frame Disabled {
      n18 = call "Pike-GetAllAttributes.vi"("Session Out 2"=w56, "error out"=w55) -> ()  [unwired: 3 out]
    }
    frame Enabled {
    }
  }
  n19 = call "IMAQdx-SetAttributes.vi"("error in"=w2, "Defaults"=T2 [{"Attribute Name"="CameraAttributes::ImageFormatControl::VideoMode", "Attribute Type"=enum."Enum", "Value"="7 = 7"}, {"Attribute Name"="CameraAttributes::ImageFormatControl::PixelFormat", "Attribute Type"=enum."Enum", "Value"="17563654  Mono 12 Packed (IIDC-msb)"}, {"Attribute Name"="CameraAttributes::AcquisitionControl::ExposureAuto", "Attribute Type"=enum."Enum", "Value"="0 = Off"}, {"Attribute Name"="AcquisitionAttributes::CameraAttributes::AcquisitionControl::AcquisitionFrameRateEnabled", "Attribute Type"=enum."Bool", "Value"="0"}], "Session Out 2"=w4) -> ("error out 2"=w1:errorcluster, "Session Out"=w3:T8)  [unwired: 1 in]
  n20 = disable-structure shown="Disabled" {
    disable-tunnel: [w64 w66] -> w22
    disable-tunnel: [w62 w65] -> w21
    disable-tunnel: w3 -> [w61 w66]
    disable-tunnel: w1 -> [w60 w65]
    frame Disabled {
      w63 = u16 0 items=["Hardware"=0, "10bit"=10, "12bit"=12, "14bit"=14, "16bit"=16]
      w59 = u32 5 items=["Mono8"=0, "Mono16"=5]  # PixelFormat
      n21 = property class="IMAQdx"(reference=w61, error in=w60, "PixelFormat"=w59, "BitsPerPixel"=w63) -> (reference out=w64:T8, error out=w62:errorcluster)
    }
    frame Enabled {
    }
  }
  n22 = Obtain Notifier(name (unnamed)="pike.number.set", notification data type=w28, error in (no error)=w18) -> (notifier out=w36:refnum<notifier>, error out=w26:errorcluster)  [unwired: 1 in, 1 out]
  n23 = Bundle("New Image"=T6 refnum, "MetaData") -> (w31:cluster{"New Image":T6, string})  [unwired: 1 out]
  n24 = Obtain Queue(max queue size (-1, unlimited)=-1, name (unnamed)="ImaqQueue", element data type=w31, create if not found? (T)=TRUE) -> (queue out=w29:refnum<queue>)  [unwired: 1 in, 2 out]
  n25 = while {
    shift-right: [w76] -> _
    shift-left: nan ("Exposure s") -> [w77]
    tunnel: w36 -> [w87]
    tunnel: w29 -> [w86]
    tunnel: [w88] -> w24
    tunnel: w21 -> [w74]
    tunnel: w26 -> [w73]
    shift-right: [w71] -> w23
    shift-left: w22 -> [w72]
    tunnel: w16 -> [w69]
    tunnel: w7 -> [w68]
    tunnel: w6 -> [w67]
    i -> [w83]
    stop <- w89 stop-if-true
    # "each Notifier"
    n26 = Wait on Notification(notifier=w87, ignore previous (F)=TRUE, error in (no error)=w73) -> (notifier out=w85:refnum<notifier>, notification=w75:string, error out=w82:errorcluster)  [unwired: 2 out]
    n27 = Unbundle By Name(w82) -> ("status"=w78:bool)
    n28 = Decimal String To Number(string=w75, default (0L)=0 ("default (0 I32)")) -> (number=w81:i32)  [unwired: 2 out]
    n29 = Less Or Equal To 0?(x=w81) -> (x <= 0?=w80:bool)
    n30 = Or(x=w80, y=w78) -> (x .or. y?=w79:bool)
    n31 = case shown="False" w79 {
      tunnel: [FALSE ("status") w225] -> w89
      tunnel: [w101 errorcluster {"status"=FALSE, "code"=0, "source"=""} ("error out")] -> w88
      tunnel: w86 -> [w128 _]
      tunnel: w85 -> [w127 _]
      tunnel: w81 -> [w125 _]
      tunnel: w78 -> [_ w225]
      tunnel: w77 -> [w124 w223]
      tunnel: [w107 w223] -> w76
      tunnel: w74 -> [w104 _]
      tunnel: w72 -> [w110 w222]
      tunnel: [w105 w222] -> w71
      tunnel: w69 -> [w96 _]
      tunnel: w68 -> [w91 _]
      tunnel: w67 -> [w90 _]
      frame False {
        # "calibration relative to IntermediateImage!"
        # "Init first time\ni need one for a preview!\nshould send sth. to metadata!"
        # "valid IMAQ!"
        # "# to do"
        # "stopp all"
        n32 = flat-sequence {
          tunnel: ["pike.save.tags" ("Tag (save.tags)")] -> w117
          tunnel: w97 -> [_]
          frame #0 {
          }
        }
        n33 = call "ImaqStorage.vi"("Command"=T10."createIMAQ") -> ("Number out"=w119:i32, "IMAQ out"=w111:T6)  [unwired: 2 in]
        n34 = call "Variables.vi"("Tag in"="pike.binning", "Command"=T4."ReadValue") -> ("value out"=w122:string)  [unwired: 1 in, 2 out]
        n35 = call "Variables.vi"("Tag in"="pike.saveall", "Command"=T4."ReadValue") -> ("value out"=w114:string)  [unwired: 1 in, 2 out]
        n36 = Decimal String To Number(string=w122, default (0L)=1 ("Standard (0 I32)")) -> (number=w108:i32)  [unwired: 2 out]
        n37 = call "GetScanMetadata.vi"("Tag (save.tags)"=w117) -> ("Metadata"=w118:string)  [unwired: 1 in, 1 out]
        n38 = case shown="\"FALSE\", Default" w114 {
          tunnel: [FALSE TRUE] -> w113
          frame "FALSE", Default {
          }
          frame "1", "TRUE" {
          }
        }
        n39 = disable-structure shown="Enabled" {
          disable-tunnel: w110 -> [w135 w138]
          disable-tunnel: [w134 w138] -> w109
          disable-tunnel: w108 -> [w133 w137]
          disable-tunnel: w104 -> [w132 w136]
          disable-tunnel: [w131 w136] -> w103
          disable-tunnel: [w130 w137] -> w95
          disable-tunnel: w91 -> [w129 _]
          frame Disabled {
            n40 = call "Pike-Binning.vi"("BinningModes"=w129, "Session In"=w135, "Binning In"=w133, "error in (no error)"=w132) -> ("Session Out"=w134:T8, "Binning Out"=w130:u32, "error out"=w131:errorcluster)  [unwired: 1 out]
          }
          frame Enabled {
          }
        }
        "binning" <- w95
        n41 = call "Calibration_ApplyBinning.vi"("magnification"=1.0, "Binning"=w95, "CalibrationCoordinates: x,x',y,y'..."=w96) -> ("CalibrationCoordinates: x,x',y,y'... 2"=w93:dbl[][])  [unwired: 1 out]
        n42 = call "2DArray_to_String.vi"("Array"=w93) -> ("String 1"=w94:string)  [unwired: 3 in, 1 out]
        n43 = call "MetaDataStorage.vi"("Number"=w119, "Meta in"=w118, "Command"=T11."saveMeta") -> ()  [unwired: 2 out]
        n44 = call "Variables.vi"("value"=w94, "Tag in"="pike.calibration", "Command"=T4."ChangeValue") -> ("value out"=w97:string)  [unwired: 2 out]
        n45 = while "nImages" {
          tunnel: w128 -> [w181]
          tunnel: w127 -> [w167]
          shift-right: [w165] -> _
          shift-left: w125 -> [w157]
          tunnel: [w148] -> w102
          shift-right: [w180] -> _
          shift-left: w111 -> [w161]
          tunnel: w113 -> [w162]
          tunnel: w109 -> [w155]
          tunnel: [w147] -> w106
          shift-right: [w152] -> w107
          shift-left: w124 -> [w171]
          tunnel: w103 -> [w151]
          tunnel: w90 -> [w145]
          i -> [w149]
          stop <- w166 continue-if-true
          w142 = u32 100  # limit to 10fps
          # "to be sure it is not U16..."
          n46 = call "Variables.vi"("Tag in"="pike.exposure", "Command"=T4."ReadValue") -> ("value out"=w174:string)  [unwired: 1 in, 2 out]
          n47 = Fract/Exp String To Number(use system decimal point (T)=FALSE, string=w174) -> (number=w154:dbl)  [unwired: 3 out]
          n48 = Not Equal?(x=w171, y=w154) -> (x != y?=w156:bool)
          n49 = case shown="True" w156 {
            tunnel: w155 -> [w183 w191]
            tunnel: w154 -> [_ w194]
            tunnel: [w183 w190] -> w153
            tunnel: w151 -> [w182 w189]
            tunnel: [w182 w188] -> w150
            tunnel: w145 -> [_ w187]
            frame False {
              # "same exposure"
            }
            frame True {
              # "max 3.2s\nFound Page67\n0-1024 : 10µs\n-1536: 20µs\n-2048: 40µs\n2560: 80µs\n-4096"
              n50 = Multiply(x=w194, y=w187) -> (x*y=w193:dbl)
              n51 = In Range and Coerce(upper limit=37000.0, x=w193, lower limit=1.0) -> (coerced(x)=w186:dbl)  [unwired: 1 out]
              n52 = property class="IMAQdx"(reference=w191, error in=w189, "ActiveAttribute"="CameraAttributes::AcquisitionControl::ExposureTime", "ValueDBL"=w186) -> (reference out=w190:T8, error out=w188:errorcluster)
            }
          }
          n53 = Equal To 0?(x=w149) -> (x = 0?=w169:bool)
          n54 = Or(x=w156, y=w169) -> (x .or. y?=w170:bool)
          n55 = case shown="True" w170 {
            tunnel: [errorcluster {"status"=FALSE, "code"=0, "source"=""} ("error out") w204] -> w160
            tunnel: w154 -> [w197 w208]
            tunnel: [w197 w208] -> w152
            tunnel: w153 -> [w196 w202]
            tunnel: [w196 w205] -> w159
            tunnel: w157 -> [_ _]
            tunnel: w150 -> [_ w198]
            frame False {
            }
            frame True {
              # "Init new image"
              n56 = call <vilib>:"IMAQdx Stop Acquisition.vi"("error in"=w198, "Session In"=w202) -> ("error out"=w200:errorcluster, "Session Out"=w201:T8)  [unwired: 8 out]
              n57 = call <vilib>:"IMAQdx Configure Acquisition.vi"("error in"=w200, "Number of Buffers"=u32 16, "Continuous?"=IMAQdx_Acquisition_Mode."Continuous", "Session In"=w201) -> ("error out"=w206:errorcluster, "Session Out"=w207:T8)  [unwired: 1 in, 5 out]
              n58 = call <vilib>:"IMAQdx Start Acquisition.vi"("error in"=w206, "Session In"=w207) -> ("error out"=w204:errorcluster, "Session Out"=w205:T8)  [unwired: 8 out]
            }
          }
          n59 = call <vilib>:"IMAQdx Get Image.vi"("Buffer Number Mode (Next)"=IMAQdx_Buffer_Number_Mode."Next", "error in"=w160, "Buffer Number In"=w149, "Image In"=w161, "Session In"=w159) -> ("error out"=w144:errorcluster, "Image Out"=w143:T6, "Session Out"=w147:T8)  [unwired: 4 out]
          n60 = call "ImaqStorage.vi"("IMAQ in"=w143, "Command"=T10."getNumber") -> ("Number out"=w163:i32)  [unwired: 1 in, 1 out]
          n61 = call "CheckContinous.vi"("notifier (var.Name / data)"=w167, "Numbers done"=w149, "Numbers to do"=w157, "error in (no error)"=w144, "Tag in (scan.number)"="pike.number" ("Tag in")) -> ("continue?"=w166:bool, "Numbers to do out"=w165:i32, "error out"=w148:errorcluster)  [unwired: 1 out]
          n62 = Number To Decimal String(number=w163) -> (decimal integer string=w178:string)  [unwired: 1 out]
          n63 = call "Variables.vi"("value"=w178, "Tag in"="pike.imaq", "Command"=T4."ChangeValue") -> ()  [unwired: 3 out]
          n64 = Not "Last"(x=w166) -> (.not. x?=w164:bool)
          n65 = Or(x=w162, y=w164) -> (x .or. y?=w179:bool)
          n66 = case shown="True" w179 {
            tunnel: w181 -> [_ w218]
            tunnel: w143 -> [w209 w211]
            tunnel: [w209 w213] -> w180
            tunnel: w164 -> [_ w212]
            frame False {
              # "last or all?"
              # "keep the IMAQ"
            }
            frame True {
              # "put into save queue\nget new one if not last run"
              n67 = call "GetScanMetadata.vi"("Tag (save.tags)"="pike.save.tags") -> ("Metadata"=w214:string)  [unwired: 1 in, 1 out]
              n68 = Concatenate Strings("name=\"pike\" " ("string"), w214) -> (w216:string)
              n69 = Bundle("Image Out"=w211, w216) -> (w215:cluster{"Image Out":T6, string})  [unwired: 1 out]
              n70 = Enqueue Element(queue=w218, element=w215) -> ()  [unwired: 1 in, 4 out]
              n71 = case shown="True" w212 {
                tunnel: [w219 w221] -> w213
                tunnel: w211 -> [_ w221]
                frame False {
                  n72 = call "ImaqStorage.vi"("Command"=T14."createIMAQ") -> ("IMAQ out"=w219:T6)  [unwired: 2 in, 1 out]
                }
                frame True {
                  # "last,\nno new IMAQ"
                }
              }
            }
          }
          n73 = Wait (ms)(milliseconds to wait=w142) -> ()  [unwired: 1 out]
          "image" <- w149
          "save all?" <- w162
        }
        n74 = call <vilib>:"IMAQdx Stop Acquisition.vi"("error in"=w102, "Session In"=w106) -> ("error out"=w101:errorcluster, "Session Out"=w105:T8)  [unwired: 8 out]
        "error" <- w101
      }
      frame True {
        # "0 images= do nothing\nerror= quit"
      }
    }
    "run" <- w83
  }
  n75 = call <vilib>:"IMAQdx Close Camera.vi"("error in"=w24, "Session In"=w23) -> ()  [unwired: 10 out]
